vi "Deadband Simple.vi"(11 "Numeric":dbl) -> (3 "t":dbl)   [LabVIEW 2016]
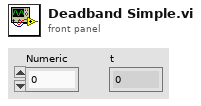
[diagram p1: front panel]
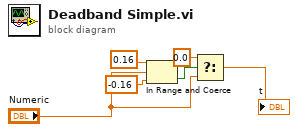
[diagram p0: block diagram]
diagram:
  n1 = In Range and Coerce(upper limit=0.16, x="Numeric", lower limit=-0.16) -> (In Range?=w4:bool)  [unwired: 1 out]
  n2 = Select(t=0.0, s=w4, f="Numeric") -> (s? t:f=→"t":dbl)
